vi "LookupError.vi"(8 "error in (no error)":errorcluster, 11 "Error info":T1) -> (0 "error out":errorcluster, 1 "Not found":bool, 2 "Log":bool, 3 "Kill":bool)   [LabVIEW 2017, in "Error.lvlib"]
doc: "Lookup the error to find shutdown mode.\nWarning if code is not found."
uses:
  Error.lvlib
  ctl/ErrorInfo.ctl
  <vilib>/Utility/config.llb/Read Key (Boolean).vi
  <vilib>/Utility/config.llb/NI_LVConfig.lvlib
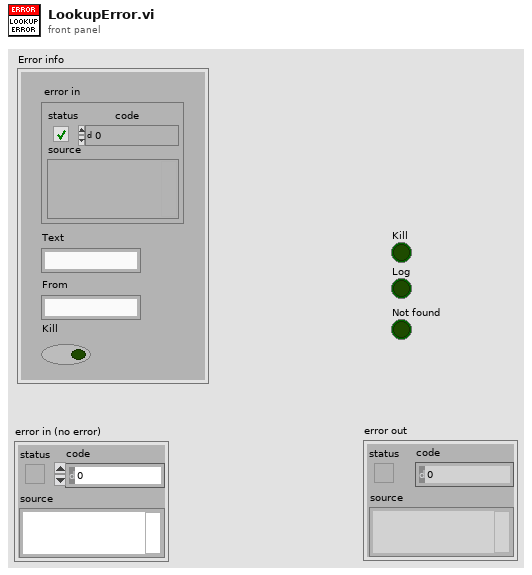
[diagram p1: front panel]
types:
  T1 = typedef "Error.lvlib/ErrorInfo.ctl" = cluster{"error in":errorcluster, "Text":string, "From":string, "Kill":bool}
  T2 = typedef "NI_LVConfig.lvlib/Config Data RefNum.ctl" = refnum<k1>
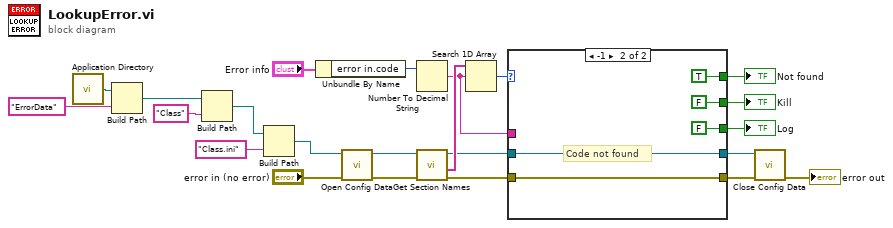
[diagram p0: block diagram]
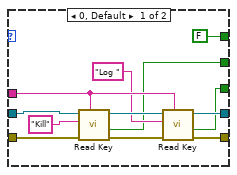
[diagram p2: hidden frame]
diagram:
  n1 = call <vilib>:"Application Directory.vi"() -> ("Application Directory"=w12:path)
  n2 = Build Path(base path=w12, name or relative path="ErrorData") -> (appended path=w10:path)
  n3 = Build Path(base path=w10, name or relative path="Class") -> (appended path=w7:path)
  n4 = Build Path(base path=w7, name or relative path="Class.ini") -> (appended path=w6:path)
  n5 = Unbundle By Name("Error info") -> ("error in.code"=w23:i32)
  n6 = call <vilib>:"Open Config Data.vi"("error in (no error)"="error in (no error)", "configuration file path"=w6) -> ("error out"=w20:errorcluster, "refnum"=w19:T2)  [unwired: 7 in, 1 out]
  n7 = Number To Decimal String(number=w23) -> (decimal integer string=w15:string)  [unwired: 1 in]
  n8 = call <vilib>:"Get Section Names.vi"("error in (no error)"=w20, "refnum"=w19) -> ("error out"=w16:errorcluster, "section names"=w18:string[], "refnum out"=w17:T2)  [unwired: 7 in]
  n9 = Search 1D Array(1D array=w18, element=w15) -> (index of element=w21:i32)  [unwired: 1 in]
  n10 = case shown="-1" w21 {
    tunnel: w17 -> [w35 w40]
    tunnel: w16 -> [w34 w39]
    tunnel: w15 -> [w31 _]
    tunnel: [w30 w40] -> w14
    tunnel: [w29 w39] -> w13
    tunnel: [w26 FALSE ("value")] -> w5
    tunnel: [w25 FALSE ("value")] -> w4
    tunnel: [FALSE ("Not found") TRUE ("Not found")] -> w1
    frame 0, Default {
      n11 = call-poly <vilib>:"Read Key.vi"("section"=w31, "error in (no error)"=w34, "key"="Kill", "refnum"=w35) -> ("error out"=w32:errorcluster, "value"=w26:bool, "refnum out"=w33:T2)  [unwired: 4 in, 1 out]
      n12 = call-poly <vilib>:"Read Key.vi"("section"=w31, "error in (no error)"=w32, "key"="Log ", "refnum"=w33) -> ("error out"=w29:errorcluster, "value"=w25:bool, "refnum out"=w30:T2)  [unwired: 4 in, 1 out]
    }
    frame -1 {
      # "Code not found"
    }
  }
  "Kill" <- w5
  "Log" <- w4
  "Not found" <- w1
  n13 = call <vilib>:"Close Config Data.vi"("error in (no error)"=w13, "refnum"=w14) -> ("error out"=→"error out":errorcluster)  [unwired: 8 in, 1 out]
